vi "onDestroyHttpSession.vi"(8 "error in (no error)":errorcluster, 11 "basic-http-client in":refnum<class "basic-http-client.lvclass">) -> (0 "error out":errorcluster, 3 "basic-http-client out":refnum<class "basic-http-client.lvclass">)   [LabVIEW 2020, in "REST Client.lvlib" / "basic-http-client.lvclass"]
uses:
  basic-http-client.lvclass
  basic-http-client.lvclass/basic-http-client.ctl
  <vilib>/httpClient/LabVIEWHTTPClient.lvlib
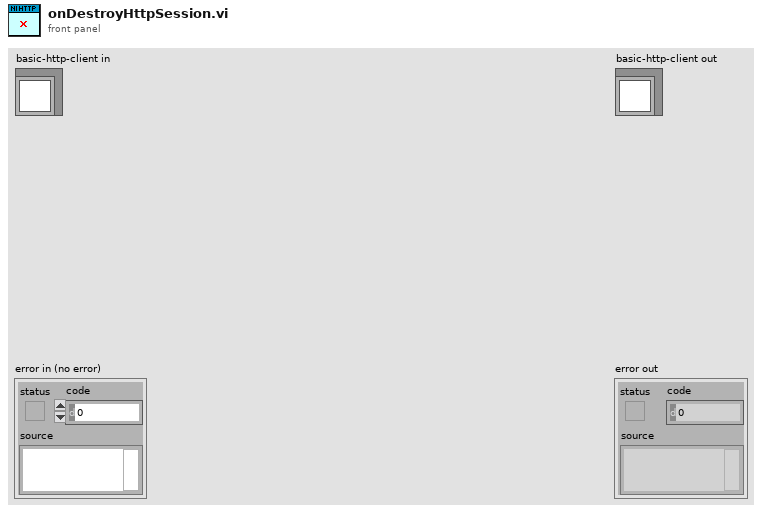
[diagram p1: front panel]
types:
  T1 = typedef "LabVIEWHTTPClient.lvlib/ClientHandle.ctl" = refnum<k1>
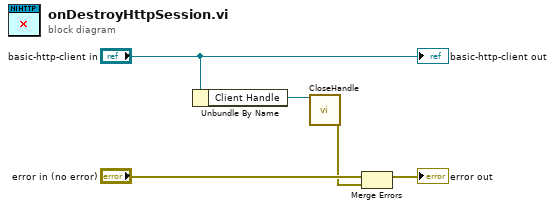
[diagram p0: block diagram]
diagram:
  n1 = Unbundle By Name("basic-http-client in") -> ("Client Handle"=w4:T1)
  n2 = call <vilib>:"CloseHandle.vi"("client handle"=w4) -> ("error out"=w1:errorcluster)  [unwired: 14 in]
  n3 = Merge Errors("error in (no error)", w1) -> (→"error out":errorcluster)
  "basic-http-client out" <- "basic-http-client in"
